vi "_PC_Pub_ExpCondi getAttributeName.vi"() -> (0 "attrName":string[](array[string]))   [LabVIEW 2018]
uses:
  RT/PublicSubVI/Ctl/_ctl_RT_ExpCondi.ctl
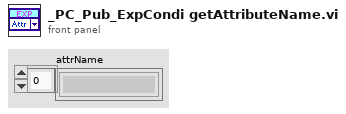
[diagram p1: front panel]
types:
  T1 = typedef "_ctl_RT_ExpCondi.ctl" = cluster{"Label":string, "Value":variant}[]
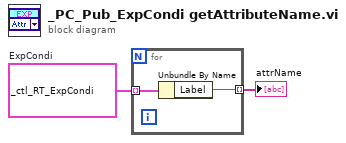
[diagram p0: block diagram]
diagram:
  w2 = T1 [{"Label"="Laser", "Value"=variant}, {"Label"="Pressure", "Value"=variant}, {"Label"="TMP", "Value"=variant}, {"Label"="Script", "Value"=variant}, {"Label"="Signal Remarks", "Value"=variant}, {"Label"="ExtAO", "Value"=variant}, {"Label"="ExtDO", "Value"=variant}, {"Label"="ExtDI", "Value"=variant}, {"Label"="D999", "Value"=variant}]  # ExpCondi
  n1 = for {
    tunnel: w2 -> [w4] mode=indexing
    tunnel: [w3] -> w1 mode=indexing
    n2 = Unbundle By Name(w4) -> ("Label"=w3:string)
  }
  "attrName" <- w1
